vi "GetCalpointNameFromID.vi"(11 "ID":T1) -> (2 "Units":string, 3 "Name":string)   [LabVIEW 2016]
uses:
  <vilib>/addons/Software Calibration Management/xSCM/Controls/ID and Element.ctl
  <vilib>/addons/Software Calibration Management/xSCM/Servers/Console-V4/CalPoint ID - V4.ctl
  <vilib>/addons/Software Calibration Management/xSCM/Controls/CalPoint - Type.ctl
  <vilib>/Utility/Data Type/NI_Data Type.lvlib
  <vilib>/addons/Software Calibration Management/xSCM/SCM-API.lvlib
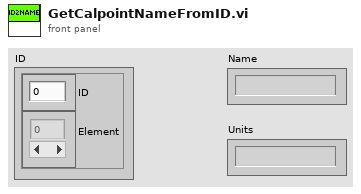
[diagram p1: front panel]
types:
  T1 = typedef "SCM-API.lvlib/ID and Element.ctl" = cluster{"ID":u32, "Element":i32[]}
  T2 = typedef "CalPoint ID - V4.ctl" = cluster{"Name":string, "Type":T3, "Control":bool, "Dimensions":u8, "Aux ID":u32, "Units":string, "Description":string, "Data Type":i16[], "Max":string, "Min":string}
  T3 = typedef "SCM-API.lvlib/CalPoint - Type.ctl" = enum8{"BOL", "U8", "U16", "U32", "U64", "I8", "I16", "I32", "I64", "SGL", "DBL", "EXT", "CSG", "CDB", "CXT", "STR", "TBL", "TLU", "CTM"}
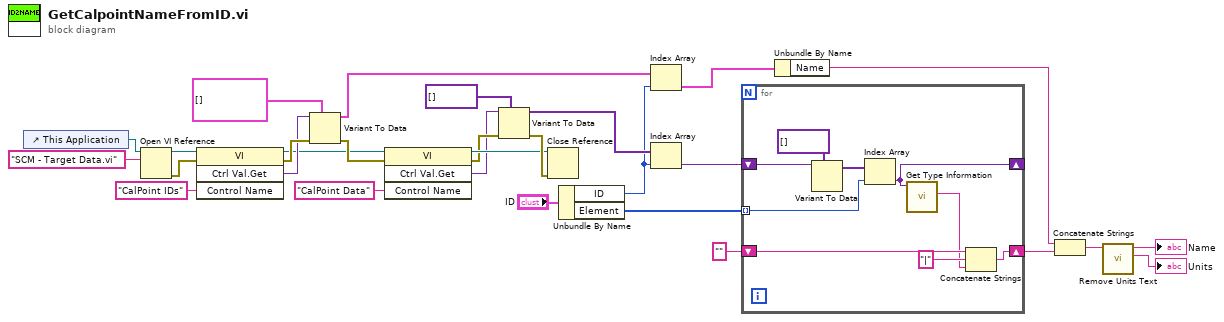
[diagram p0: block diagram]
diagram:
  n1 = control-ref of="This Application"() -> (w5:refnum<vi>)
  n2 = Open VI Reference(application reference (local)=w5, vi path="SCM - Target Data.vi") -> (vi reference=w14:refnum<vi>, error out=w18:errorcluster)  [unwired: 4 in]
  n3 = invoke class="VI" method="Ctrl Val.Get"(reference=w14, error in=w18, "Control Name"="CalPoint IDs") -> (reference out=w16:refnum<vi>, error out=w21:errorcluster, "Get Control Value Variant"=w19:variant)  [unwired: 1 in, 1 out]
  n4 = Variant To Data(error in=w21, type=T2[] [] ("CalPoint IDs"), Variant=w19) -> (data=w26:T2[], error out=w22:errorcluster)
  n5 = invoke class="VI" method="Ctrl Val.Get"(reference=w16, error in=w22, "Control Name"="CalPoint Data") -> (reference out=w28:refnum<vi>, error out=w23:errorcluster, "Get Control Value Variant"=w20:variant)  [unwired: 1 in, 1 out]
  n6 = Variant To Data(error in=w23, type=variant[] [] ("CalPoint Data"), Variant=w20) -> (data=w27:variant[], error out=w29:errorcluster)
  n7 = Close Reference(reference=w28, error in (no error)=w29) -> ()  [unwired: 1 out]
  n8 = Unbundle By Name("ID") -> ("ID"=w11:u32, "Element"=w10:i32[])
  n9 = Index Array(array=w26, index=w11) -> (element=w12:T2)
  n10 = Index Array(array=w27, index=w11) -> (element=w8:variant)
  n11 = for {
    tunnel: w10 -> [w35] mode=indexing
    shift-right: [w34] -> _
    shift-left: w8 -> [w37]
    shift-right: [w30] -> w4
    shift-left: "" ("Name") -> [w33]
    n12 = Variant To Data(type=variant[] [], Variant=w37) -> (data=w36:variant[])  [unwired: 1 in, 1 out]
    n13 = Index Array(array=w36, index=w35) -> (element=w34:variant)
    n14 = call <vilib>:"Get Type Information.vi"("Variant"=w34) -> ("Name"=w31:string)  [unwired: 6 in, 4 out]
    n15 = Concatenate Strings(w33, "|" ("Name"), w31) -> (w30:string)
  }
  n16 = Unbundle By Name(w12) -> ("Name"=w6:string)
  n17 = Concatenate Strings(w6, w4) -> (w3:string)
  n18 = call <vilib>:"Remove Units Text.vi"("Name"=w3) -> ("Units"=→"Units":string, "Name"=→"Name":string)  [unwired: 9 in]
